vi "investigate_sig.vi"() -> ()   [LabVIEW 2025]
panel:
  out "size(s)":i32[](array[numeric])
  out "Signals":dynamicdata(graph)
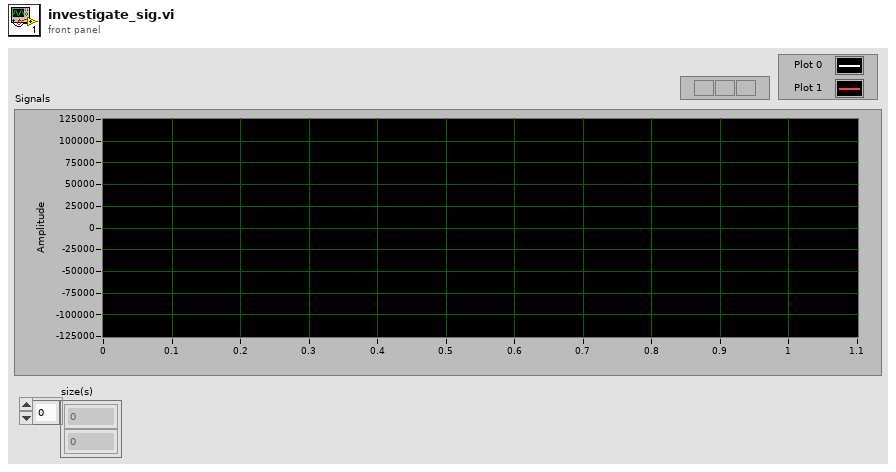
[diagram p1: front panel]
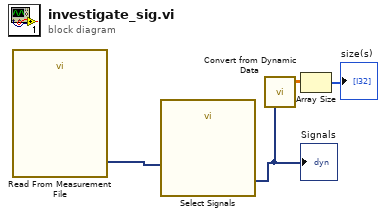
[diagram p0: block diagram]
diagram:
  n1 = call "Read From Measurement File"() -> ("Signals"=w4:dynamicdata)  [unwired: 6 in, 5 out]
  n2 = call "Select Signals"("Signals"=w4) -> ("Signal Out"=w3:dynamicdata)  [unwired: 9 in, 1 out]
  "Signals" <- w3
  n3 = call "Convert from Dynamic Data"("Dynamic Data Type"=w3) -> ("Array"=w2:dbl[][])  [unwired: 3 in]
  n4 = Array Size(array=w2) -> (size(s)=→"size(s)":i32[])
